vi "Strain_Test.vi"() -> ()   [LabVIEW 2020]
uses:
  vi.lib/Utility/TradDaqScaling.llb/Convert Strain Gauge Reading (scaler).vi
panel:
  out "Strain":sgl format="%0.6f"
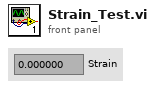
[diagram p1: front panel]
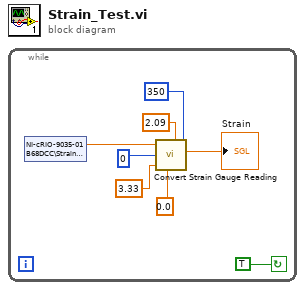
[diagram p0: block diagram]
diagram:
  n1 = while {
    stop <- TRUE continue-if-true
    n2 = shared-variable "NI-cRIO-9035-01B68DCC\\Strain Gauge\\AI1"() -> (w1:dbl)  [unwired: 1 in, 1 out]
    n3 = call-poly "Convert Strain Gauge Reading.vi"("Vsg (0.0)"=w1, "Bridge Configuration\n(3:Half Bridge II)"=0, "Vex (3.33)"=3.33, "Vinit (0.0)"=0.0, "GF (2.0)"=2.09, "Rg (120)"=350) -> ("Strain"=→"Strain":sgl)  [unwired: 4 in]
  }
